vi "Mecanum Control.vi"(11 "Drive Controls":T1) -> (3 "Wheel m's":cluster{dbl, dbl, dbl, dbl})   [LabVIEW 2014]
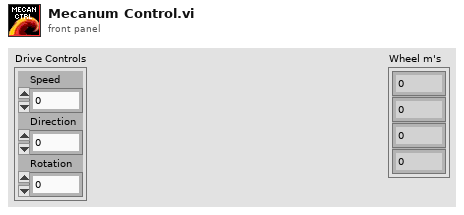
[diagram p1: front panel]
types:
  T1 = cluster{"Speed":dbl, "Direction":dbl, "Rotation":dbl}
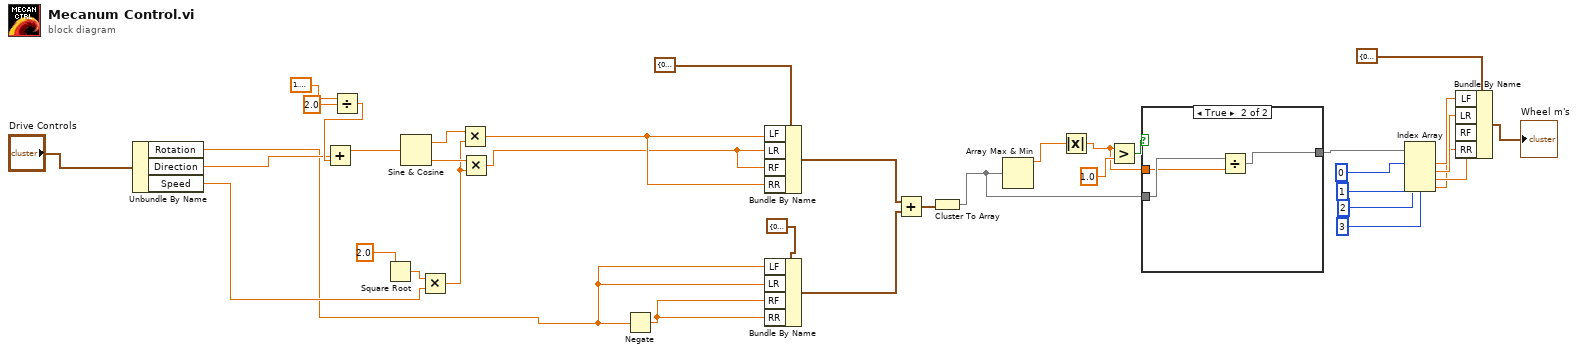
[diagram p0: block diagram]
diagram:
  n1 = Unbundle By Name("Drive Controls") -> ("Rotation"=w2:dbl, "Direction"=w4:dbl, "Speed"=w3:dbl)
  n2 = Divide(x=1.5707963267948966 ("y"), y=2.0) -> (x/y=w24:dbl)
  n3 = Add(x=w4, y=w24) -> (x+y=w30:dbl)
  n4 = Square Root(x=2.0) -> (sqrt(x)=w28:dbl)
  n5 = Sine & Cosine(0:w30) -> (1:w36:dbl, 2:w37:dbl)
  n6 = Multiply(x=w28, y=w3) -> (x*y=w27:dbl)
  n7 = Multiply(x=w36, y=w27) -> (x*y=w23:dbl)
  n8 = Multiply(x=w37, y=w27) -> (x*y=w22:dbl)
  n9 = Negate(x=w2) -> (-x=w31:dbl)
  n10 = Bundle By Name(cluster=cluster{"LF":dbl, "LR":dbl, "RF":dbl, "RR":dbl} {"LF"=0.0, "LR"=0.0, "RF"=0.0, "RR"=0.0} ("Motor Powers"), "LF"=w23, "LR"=w22, "RF"=w22, "RR"=w23) -> (w33:cluster{"LF":dbl, "LR":dbl, "RF":dbl, "RR":dbl})
  n11 = Bundle By Name(cluster=cluster{"LF":dbl, "LR":dbl, "RF":dbl, "RR":dbl} {"LF"=0.0, "LR"=0.0, "RF"=0.0, "RR"=0.0} ("Motor Powers 2"), "LF"=w2, "LR"=w2, "RF"=w31, "RR"=w31) -> (w32:cluster{"LF":dbl, "LR":dbl, "RF":dbl, "RR":dbl})
  n12 = Add(x=w33, y=w32) -> (x+y=w21:cluster{"LF":dbl, "LR":dbl, "RF":dbl, "RR":dbl})
  n13 = Cluster To Array(cluster=w21) -> (array=w17:dbl[])
  n14 = Array Max & Min(array=w17) -> (max value=w20:dbl)  [unwired: 3 out]
  n15 = Absolute Value(x=w20) -> (abs(x)=w16:dbl)
  n16 = Greater?(x=w16, y=1.0) -> (0:w18:bool)
  n17 = case shown="True" w18 {
    tunnel: w17 -> [w38 w41]
    tunnel: w16 -> [_ w40]
    tunnel: [w38 w39] -> w14
    frame False {
    }
    frame True {
      n18 = Divide(x=w41, y=w40) -> (x/y=w39:dbl[])
    }
  }
  n19 = Index Array(array=w14, index #1=0 ("index"), index #2=1 ("index"), index #3=2 ("index"), index #4=3 ("index")) -> (element #1=w15:dbl, element #2=w12:dbl, element #3=w11:dbl, element #4=w10:dbl)
  n20 = Bundle By Name(cluster=cluster{"LF":dbl, "LR":dbl, "RF":dbl, "RR":dbl} {"LF"=0.0, "LR"=0.0, "RF"=0.0, "RR"=0.0} ("Motor Powers"), "LF"=w15, "LR"=w12, "RF"=w11, "RR"=w10) -> (→"Wheel m's":cluster{"LF":dbl, "LR":dbl, "RF":dbl, "RR":dbl})
